vi "建造者模式DEMO.vi"() -> ()   [LabVIEW 2013]
uses:
  Director_class/Director.lvclass
  Gear_class/Gear.lvclass
  Cylinder_class/Cylinder.lvclass
  <vilib>/addons/_AddQ/G#Object/G#Object.lvclass
panel:
  in  "停止":bool
  in  "生产油缸":bool
  in  "生产齿轮":bool
  out "Output":string
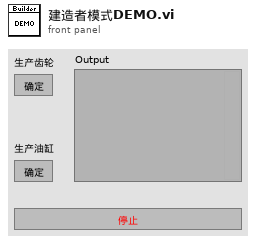
[diagram p1: front panel]
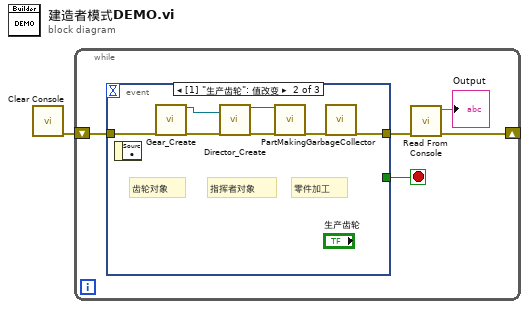
[diagram p0: block diagram]
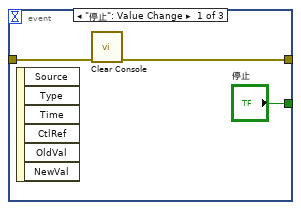
[diagram p2: hidden frame]
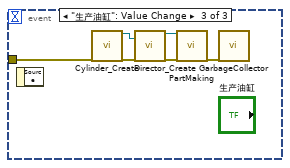
[diagram p3: hidden frame]
diagram:
  n1 = call "Clear Console.vi"() -> ("error out"=w1:errorcluster)  [unwired: 11 in]
  n2 = while {
    shift-right: [w2] -> _
    shift-left: w1 -> [w5]
    stop <- w6 stop-if-true
    n3 = event shown="[1] \"生产齿轮\": 值改变" {
      selector: _ -> [_ _ _]
      dyn-events: _ -> [_ _ _]
      timeout: _ -> [_ _ _]
      tunnel: ["停止" _ _] -> w6
      tunnel: w5 -> [w8 w10 w20]
      tunnel: [w7 w11 _] -> w3
      event "停止": Value Change {
        n4 = event-data() -> ()  [unwired: 1 in, 6 out]
        n5 = call "Clear Console.vi"("error in (no error)"=w8) -> ("error out"=w7:errorcluster)  [unwired: 10 in]
      }
      event "生产齿轮": Value Change {
        # "零件加工"
        # "指挥者对象"
        # "齿轮对象"
        n6 = event-data() -> ()  [unwired: 1 in, 1 out]
        n7 = call "Gear_Create.vi"("error in (no error)"=w10) -> ("reference out"=w13:refnum<class "Gear.lvclass">, "error out"=w14:errorcluster)  [unwired: 17 in]
        n8 = call "Director_Create.vi"("Part.lvclass"=w13, "error in (no error)"=w14) -> ("reference out"=w15:refnum<class "Director.lvclass">, "error out"=w16:errorcluster)  [unwired: 16 in]
        n9 = call-dynamic "PartMaking.vi"("reference in"=w15, "error in (no error)"=w16) -> ("error out"=w12:errorcluster)  [unwired: 16 in, 1 out]
        n10 = call <vilib>:"GarbageCollector.vi"("error in (no error)"=w12) -> ("error out"=w11:errorcluster)  [unwired: 16 in, 2 out]
      }
      event "生产油缸": Value Change {
        n11 = event-data() -> ()  [unwired: 1 in, 1 out]
        n12 = call "Cylinder_Create.vi"("error in (no error)"=w20) -> ("reference out"=w18:refnum<class "Cylinder.lvclass">, "error out"=w19:errorcluster)  [unwired: 17 in]
        n13 = call "Director_Create.vi"("Part.lvclass"=w18, "error in (no error)"=w19) -> ("reference out"=w17:refnum<class "Director.lvclass">, "error out"=w22:errorcluster)  [unwired: 16 in]
        n14 = call-dynamic "PartMaking.vi"("reference in"=w17, "error in (no error)"=w22) -> ("error out"=w21:errorcluster)  [unwired: 16 in, 1 out]
        n15 = call <vilib>:"GarbageCollector.vi"("error in (no error)"=w21) -> ()  [unwired: 16 in, 3 out]
      }
    }
    n16 = call "Read From Console.vi"("error in (no error)"=w3) -> ("error out"=w2:errorcluster, "Output"=→"Output":string)  [unwired: 9 in]
  }
